vi "Handle Drag.vi"(7 "Done? (F)":bool, 9 "Available Data Names":string[](array[string]), 10 "Coords":T1, 11 "SequenceViewPanel in":refnum<class "SequenceViewPanel.lvclass">) -> (1 "Index":i32, 2 "Step Type Name":string, 3 "SequenceViewPanel out":refnum<class "SequenceViewPanel.lvclass">, 4 "Accepted?":bool)   [LabVIEW 2020, in "TSnax UI.lvlib" / "SequenceViewPanel.lvclass"]
uses:
  SequenceViewPanel.lvclass
  <vilib>/Utility/miscctls.llb/LVPoint32TypeDef.ctl
  Drag Data Names.ctl
  SequenceViewPanel.lvclass/SequenceViewPanel.ctl
  52703bb3-bc71-497d-a9d4-2f3dd9cc266b.vi
  11c460cf-3c17-418e-a9ab-802b58c45a96.vi
  <vilib>/Comparison/Equal/Equal Functor/Equal Functor.lvclass
  TSnax UI.lvlib
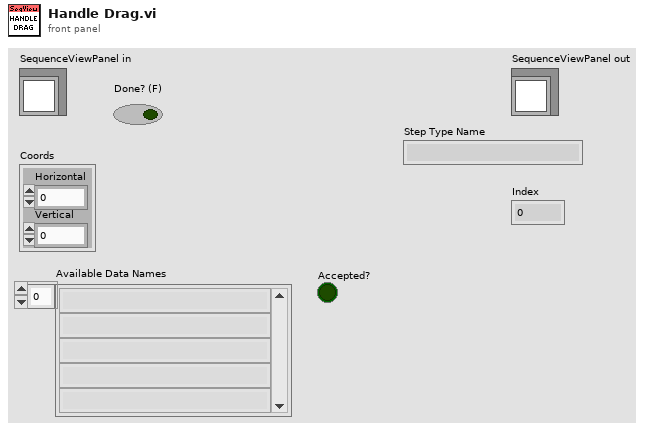
[diagram p1: front panel]
types:
  T1 = typedef "LVPoint32TypeDef.ctl" = cluster{"Horizontal":i32, "Vertical":i32}
  T2 = typedef "TSnax UI.lvlib/Drag Data Names.ctl" = enum16{"TSnax_InsertStep"}
  T3 = typedef "TSnax UI.lvlib/SequenceViewPanel.lvclass/Ref Data.ctl" = cluster{"Insert Index":i32}
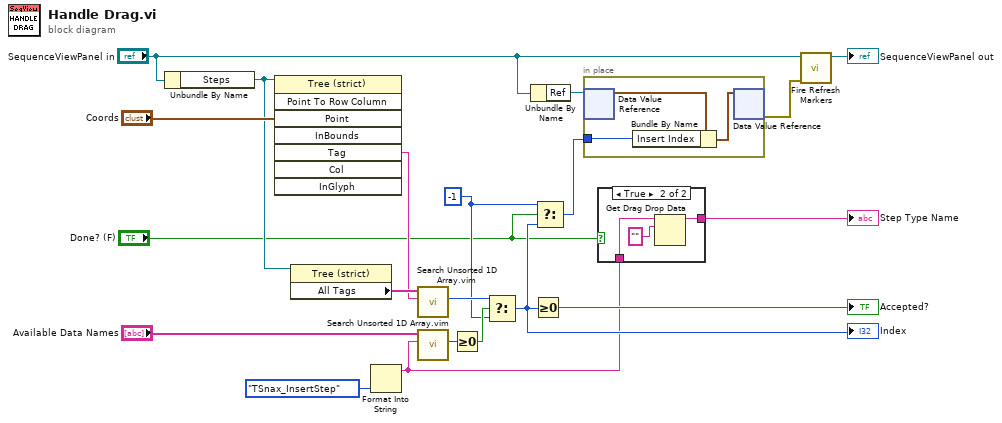
[diagram p0: block diagram]
diagram:
  w5 = -1 ("f")
  n1 = Unbundle By Name("SequenceViewPanel in") -> ("Steps"=w10:refnum<vi>)
  n2 = invoke on="Invoke Node" class="Tree (strict)" method="Point To Row Column"(reference=w10, "Point"="Coords") -> ("Tag"=w19:string)  [unwired: 6 in, 7 out]
  n3 = property on="Property Node" class="Tree (strict)"(reference=w10) -> ("All Tags"=w20:string[])  [unwired: 1 in, 2 out]
  n4 = Format Into String(Drag_Data_Names."TSnax_InsertStep" ("Drag Data Names")) -> (resulting string=w2:string)  [unwired: 3 in, 1 out]
  n5 = call "Search Unsorted 1D Array.vim"("element"=w19, "unsorted 1D array"=w20) -> ("index of element"=w15:i32)  [unwired: 9 in]
  n6 = call "Search Unsorted 1D Array.vim"("element"=w2, "unsorted 1D array"="Available Data Names") -> ("index of element"=w16:i32)  [unwired: 9 in]
  n7 = Greater Or Equal To 0?(x=w16) -> (x >= 0?=w14:bool)
  n8 = Select(t=w15, s=w14, f=w5) -> (s? t:f=w6:i32)
  "Index" <- w6
  n9 = Unbundle By Name("SequenceViewPanel in") -> ("Ref"=w18:refnum<data-value>)
  n10 = Greater Or Equal To 0?(x=w6) -> (x >= 0?=→"Accepted?":bool)
  n11 = Select(t=w5, s="Done? (F)", f=w6) -> (s? t:f=w4:i32)
  n12 = in-place {
    in-place-border: w4 -> [w21]
    n13 = in-place-dvr #1(w18) -> (w23:T3)  [unwired: 1 out]
    n14 = Bundle By Name(cluster=w23, "Insert Index"=w21) -> (w22:T3)
    n15 = in-place-dvr #1(w22) -> (w7:errorcluster)  [unwired: 1 out]
  }
  n16 = case shown="True" "Done? (F)" {
    tunnel: w2 -> [_ w25]
    tunnel: [_ w24] -> w1
    frame False {
    }
    frame True {
      n17 = Get Drag Drop Data(8:"", 9:w25) -> (3:w24:string)  [unwired: 1 in, 1 out]
    }
  }
  "Step Type Name" <- w1
  n18 = call "Fire Refresh Markers.vi"("error in (no error)"=w7, "SequenceViewPanel in"="SequenceViewPanel in") -> ("SequenceViewPanel out"=→"SequenceViewPanel out":refnum<class "SequenceViewPanel.lvclass">)  [unwired: 8 in, 1 out]
